vi "CfgManager Cache Lifetime Tests.vi"() -> ()   [LabVIEW 2013]
uses:
  Manager/ConfigManager.lvclass
  Collection/ConfigManagerCollection.lvclass
  Cache/ConfigManager.Cache.lvclass
panel:
  out "Values":variant[](array[variant])
  out "Keys 2":string[](array[string])
  out "Keys":string[](array[string])
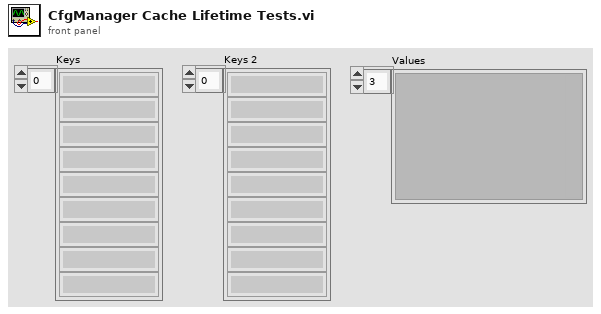
[diagram p1: front panel]
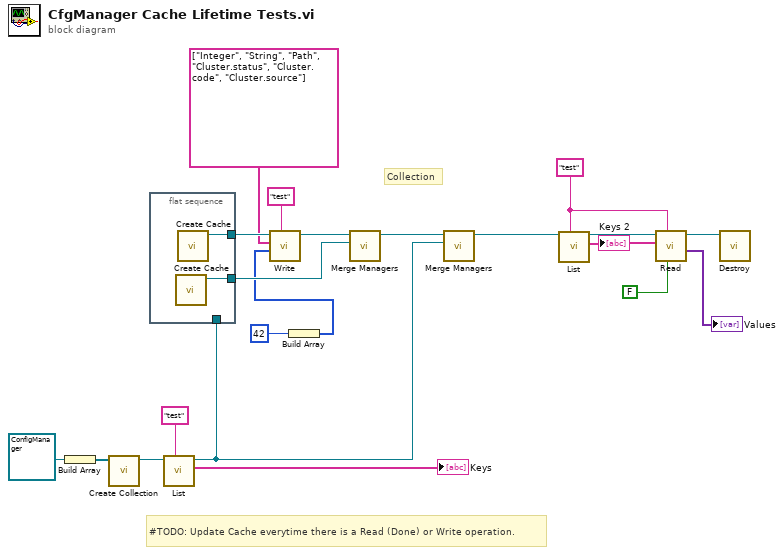
[diagram p0: block diagram]
diagram:
  w8 = "test" ("Qualified Name")
  # "#TODO: Update Cache everytime there is a Read (Done) or Write operation."
  # "Collection"
  n1 = Build Array(refnum<class "ConfigManager.lvclass"> refnum ("SMOConfig.lvlib:ConfigManager.lvclass")) -> (w17:refnum<class "ConfigManager.lvclass">[])
  n2 = call "Create Collection.vi"("List"=w17) -> ("SMOConfigManagerCollection out"=w16:refnum<class "ConfigManagerCollection.lvclass">)  [unwired: 10 in]
  n3 = flat-sequence {
    tunnel: [w23] -> w21
    tunnel: [w22] -> w19
    tunnel: w15 -> [_]
    frame #0 {
      n4 = call "Create Cache.vi"() -> ("ConfigManager.Cache"=w23:refnum<class "ConfigManager.Cache.lvclass">)  [unwired: 11 in]
      n5 = call "Create Cache.vi"() -> ("ConfigManager.Cache"=w22:refnum<class "ConfigManager.Cache.lvclass">)  [unwired: 11 in]
    }
  }
  n6 = call "List.vi"("Qualified Name"="test", "ConfigManager in"=w16) -> ("Keys"=→"Keys":string[], "ConfigManager out"=w15:refnum<class "ConfigManagerCollection.lvclass">)  [unwired: 7 in, 1 out]
  n7 = Build Array(42) -> (w5:i32[])
  n8 = call "Write.vi"("Qualified Name"="test", "Values"=w5, "keys"=string[] ["Integer", "String", "Path", "Cluster.status", "Cluster.code", "Cluster.source"], "ConfigManager in"=w19) -> ("ConfigManager out"=w3:refnum<class "ConfigManager.Cache.lvclass">)  [unwired: 5 in, 2 out]
  n9 = call "Merge Managers.vi"("ConfigManager B"=w21, "ConfigManager A"=w3) -> ("ConfigManagerCollection"=w20:refnum<class "ConfigManagerCollection.lvclass">)  [unwired: 9 in]
  n10 = call "Merge Managers.vi"("ConfigManager B"=w15, "ConfigManager A"=w20) -> ("ConfigManagerCollection"=w2:refnum<class "ConfigManagerCollection.lvclass">)  [unwired: 9 in]
  n11 = call "List.vi"("Qualified Name"=w8, "ConfigManager in"=w2) -> ("Keys"=w7:string[], "ConfigManager out"=w10:refnum<class "ConfigManagerCollection.lvclass">)  [unwired: 7 in, 1 out]
  "Keys 2" <- w7
  n12 = call "Read.vi"("prioritize Cache? (F)"=FALSE ("use Cache? (F)"), "Qualified Name"=w8, "keys in"=w7, "ConfigManager in"=w10) -> ("Values"=→"Values":variant[], "ConfigManager out"=w9:refnum<class "ConfigManagerCollection.lvclass">)  [unwired: 4 in, 2 out]
  n13 = call-dynamic "Destroy.vi"("ConfigManagerCollection in"=w9) -> ()  [unwired: 9 in, 2 out]
